vi "Get Configuration Settings Config.vi"(8 "error in (no error)":errorcluster) -> (0 "error out":errorcluster, 2 "Configuration":T1={"Samples per Read"=0, "Number of Reads to Save"=0, "Data File Name"="", "TDMS Properties"=[], "Number of Channels"=4, "Trigger - RMS Value"=0.0, "Trigger - Channel"=0, "Trigger - Time (Minute)"=0, "Channel Config"=[], "data rate (S/s)"=0, "Time Measure"=0.0} {"Channel Config"."Input Configuration" items=["AC Coupled", "DC Coupled", "IEPE AC Coupled"]})   [LabVIEW 2015]
uses:
  Acquisition and Logging Configuration_Waveform.ctl
  TDMS Properties.ctl
  <vilib>/LabVIEW Targets/FPGA/cRIO/shared/nicrio_ModuleControls/nicrio_cRIO-9234_ConfigModeRing.ctl
  <vilib>/Utility/xml.llb/Read From XML File(string).vi
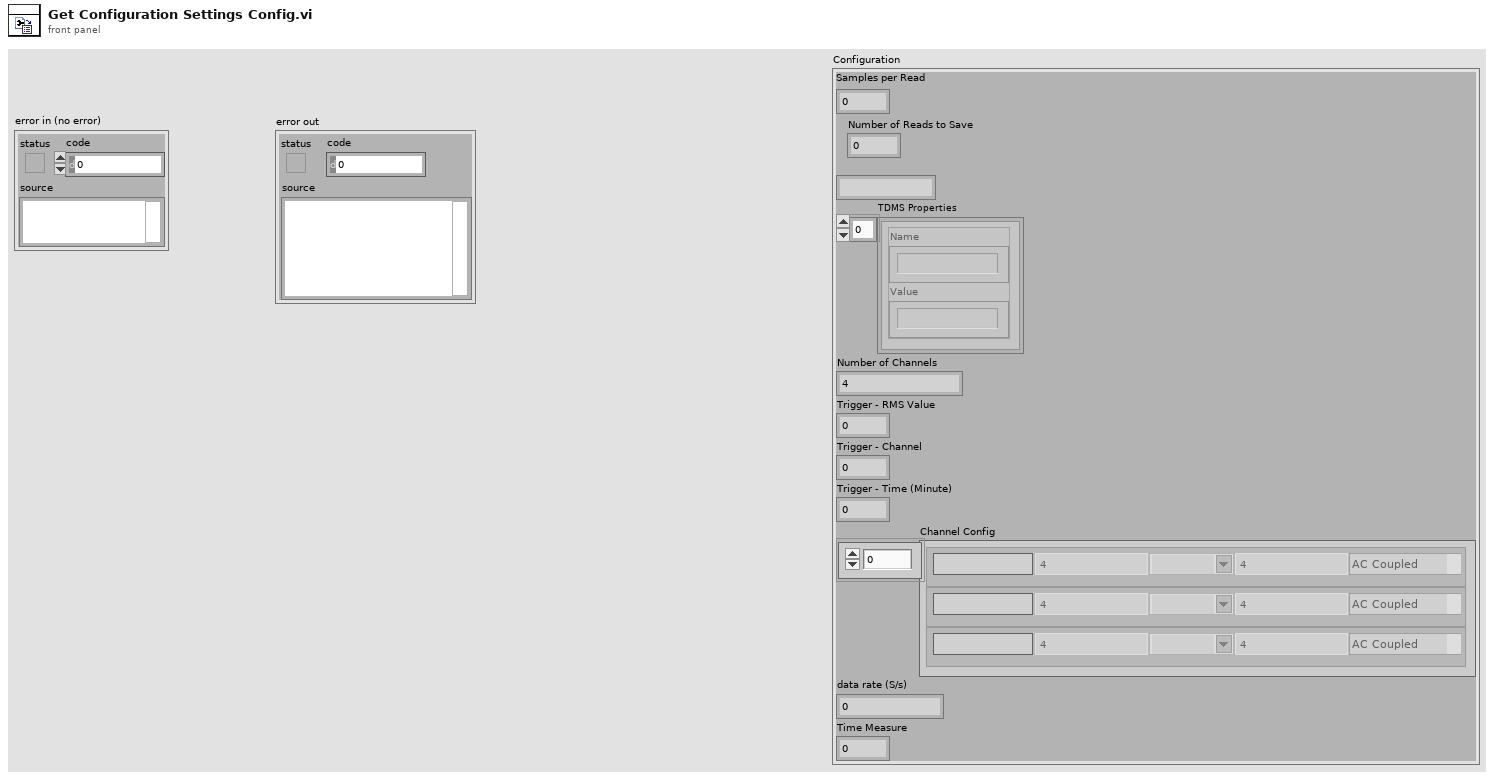
[diagram p1: front panel]
types:
  T1 = typedef "Acquisition and Logging Configuration_Waveform.ctl" = cluster{"Samples per Read":i32, "Number of Reads to Save":i32, "Data File Name":string, "TDMS Properties":T2[], "Number of Channels":i32, "Trigger - RMS Value":dbl, "Trigger - Channel":i32, "Trigger - Time (Minute)":i32, "Channel Config":cluster{"Channel Name":string, "Sensitivity mV_EU":dbl, "EU":string, "Input Configuration":T3, "dB Ref EU":dbl}[], "data rate (S/s)":u32, "Time Measure":dbl}
  T2 = typedef "TDMS Properties.ctl" = cluster{"Name":string, "Value":string}
  T3 = typedef "nicrio_cRIO-9234_ConfigModeRing.ctl" = u8
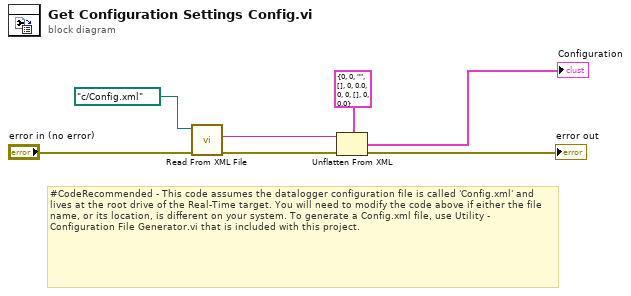
[diagram p0: block diagram]
diagram:
  # "#CodeRecommended - This code assumes the datalogger configuration file is called 'Config.xml' and lives at the root drive of the Real-Time target. You will need to modify the code above if either the file name, or its location, is different on your system. To generate a Config.xml file, use Utility - Configuration File Generator.vi that is included with this project."
  n1 = call-poly <vilib>:"Read From XML File.vi"("error in (no error)"="error in (no error)", "XML File Path"=path "c:/Config.xml") -> ("error out"=w6:errorcluster, "XML Elements"=w5:string)  [unwired: 7 in, 1 out]
  n2 = Unflatten From XML(xml string=w5, type=T1 {"Samples per Read"=0, "Number of Reads to Save"=0, "Data File Name"="", "TDMS Properties"=[], "Number of Channels"=0, "Trigger - RMS Value"=0.0, "Trigger - Channel"=0, "Trigger - Time (Minute)"=0, "Channel Config"=[], "data rate (S/s)"=0, "Time Measure"=0.0} ("VibLog Configuration"), error in (no error)=w6) -> (value=→"Configuration":T1, error out=→"error out":errorcluster)
